vi "Windows Simulate 5 Wire xVDT.vi"() -> ()   [LabVIEW 2011]
uses:
  <vilib>/ptbypt/NI_PtbyPt.lvlib
panel:
  in  "Stimulus Volts":i16=10
  out "(Va-Vb)/(Va+Vb)":dbl
  out "Va+Vb/2":dbl
  out "Vb RMS":dbl format="%0.2f"
  out "Va RMS":dbl format="%0.2f"
  out "Stim RMS":dbl format="%0.2f"
  out "LVDT 2":dynamicdata(graph)
  in  "Transfer Ratio(V/V)":dbl=0.6
  in  "Scaling Factor 2":fxp<+/-,19,5>
  out "LVDT":dynamicdata(graph)
  in  "Position (mm)":dbl(slide) caption="Position" scale=-8.0..8.0 scale format="%.2f"
  in  "Difference over sum gain":dbl=0.045
  in  "stop":bool
  in  "Scaling Factor 1":fxp<+/-,19,5>
  # "Setup"
  # "Run-Time"
  # "Display"
  # "Transfer Ratio or Sum Ratio = (Va+Vb)/Ve"
  # "Difference over sum gain = ((Va-Vb)/(Va+Vb))/d"
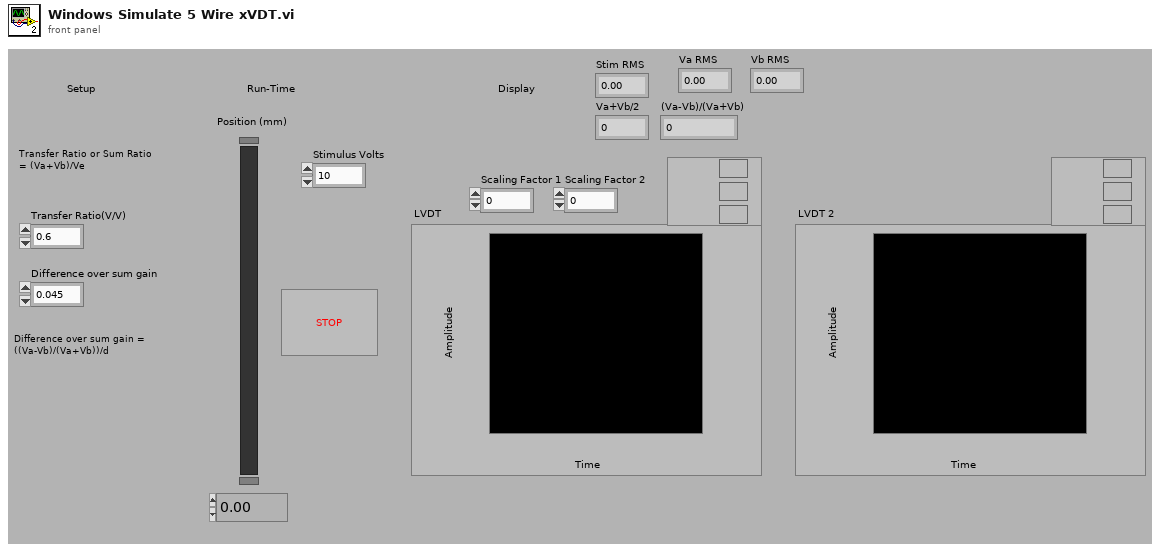
[diagram p1: front panel]
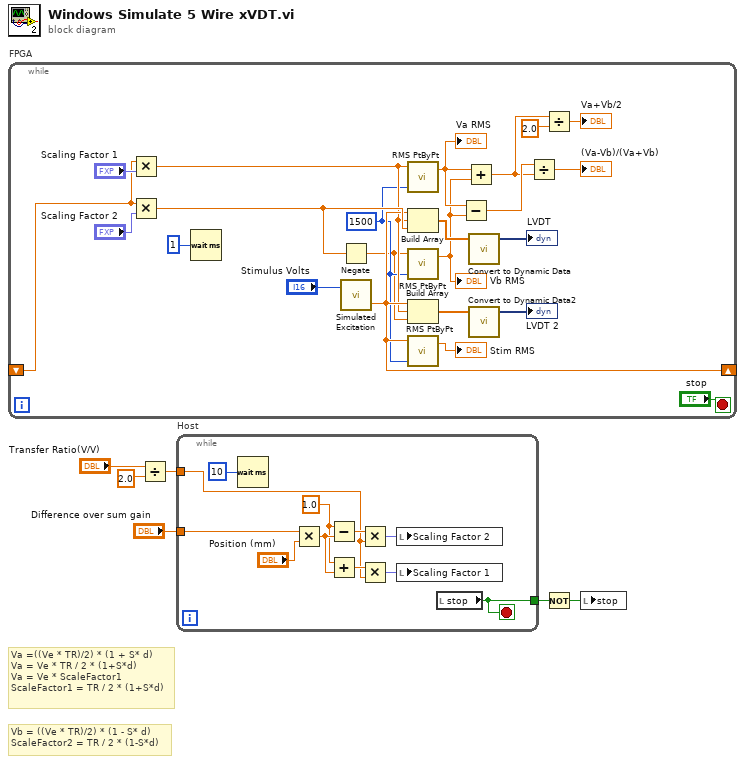
[diagram p0: block diagram]
diagram:
  # "Vb = ((Ve * TR)/2) * (1 - S* d)\nScaleFactor2 = TR / 2 * (1-S*d)"
  # "Va =((Ve * TR)/2) * (1 + S* d)\nVa = Ve * TR / 2 * (1+S*d)\nVa = Ve * ScaleFactor1\nScaleFactor1 = TR / 2 * (1+S*d)"
  n1 = while "FPGA" {
    shift-right: [w19] -> _
    shift-left: _ -> [w23]
    stop <- "stop" stop-if-true
    w16 = 1500 ("sample length")
    n2 = Multiply(x=w23, y="Scaling Factor 1") -> (x*y=w17:dbl)
    n3 = Multiply(x=w23, y="Scaling Factor 2") -> (x*y=w21:dbl)
    n4 = Wait (ms)(milliseconds to wait=u32 1) -> ()  [unwired: 1 out]
    n5 = Negate(x=w21) -> (-x=w15:dbl)
    n6 = call "Simulated Excitation.vi"("Volts"="Stimulus Volts") -> ("Analog Input"=w19:dbl)  [unwired: 2 in]
    n7 = call <vilib>:"RMS PtByPt.vi"("sample length"=w16, "x"=w17) -> ("rms value"=w12:dbl)  [unwired: 2 in, 1 out]
    "Va RMS" <- w12
    n8 = Build Array(w19, w17, w21) -> (w28:dbl[])
    n9 = call <vilib>:"RMS PtByPt.vi"("sample length"=w16, "x"=w15) -> ("rms value"=w11:dbl)  [unwired: 2 in, 1 out]
    "Vb RMS" <- w11
    n10 = Build Array(w19, w17, w15) -> (w22:dbl[])
    n11 = call <vilib>:"RMS PtByPt.vi"("sample length"=w16, "x"=w19) -> ("rms value"=→"Stim RMS":dbl)  [unwired: 2 in, 1 out]
    n12 = Subtract(x=w12, y=w11) -> (x-y=w10:dbl)
    n13 = Add(x=w12, y=w11) -> (x+y=w9:dbl)
    n14 = call "Convert to Dynamic Data"("Array"=w28) -> ("Dynamic Data Type"=→"LVDT":dynamicdata)  [unwired: 3 in]
    n15 = call "Convert to Dynamic Data2"("Array"=w22) -> ("Dynamic Data Type"=→"LVDT 2":dynamicdata)  [unwired: 3 in]
    n16 = Divide(x=w10, y=w9) -> (x/y=→"(Va-Vb)/(Va+Vb)":dbl)
    n17 = Divide(x=w9, y=2.0) -> (x/y=→"Va+Vb/2":dbl)
  }
  n18 = Divide(x="Transfer Ratio(V/V)", y=2.0 ("x")) -> (x/y=w3:dbl)
  n19 = while "Host" {
    tunnel: "Difference over sum gain" -> [w38]
    tunnel: w3 -> [w31]
    tunnel: [w30] -> w1
    stop <- w30 stop-if-true
    w32 = 1.0 ("x")
    n20 = Wait (ms)(milliseconds to wait=u32 10) -> ()  [unwired: 1 out]
    n21 = Multiply(x=w38, y="Position (mm)") -> (x*y=w37:dbl)
    n22 = Subtract(x=w32, y=w37) -> (x-y=w36:dbl)
    n23 = Add(x=w32, y=w37) -> (x+y=w35:dbl)
    n24 = Multiply(x=w36, y=w31) -> (x*y=w33:fxp<+/-,19,5>)
    n25 = Multiply(x=w35, y=w31) -> (x*y=w34:fxp<+/-,19,5>)
    n26 = local write "Scaling Factor 2"(w33) -> ()
    n27 = local write "Scaling Factor 1"(w34) -> ()
    n28 = local read "stop"() -> (w30:bool)
  }
  n29 = Not(x=w1) -> (.not. x?=w6:bool)
  n30 = local write "stop"(w6) -> ()
